vi "XImc Example One axis.vi"() -> ()   [LabVIEW 2017]
uses:
  subvi/XImc Example 1 CS.ctl
  libximc.lvlib
panel:
  in  "?":enum32{"Move settings"}(tab)
  in  "Speed":i32
  in  "GMOV":bool
  in  "SMOV":bool
  in  "Accel":i32
  in  "Decel":i32
  in  "Antiplay":i32
  out "Speed":dbl format="%#.2f"
  out "Accel":i16
  out "Decel":i16 format="%#.2f"
  out "Antiplay":i32
  out "Speed":dbl format="%#.2f steps/s"
  out "Temperature":dbl format="%#.2f C"
  out "USB current":dbl format="%#.2f mA"
  out "USB voltage":dbl format="%#.2f V"
  out "Power current":dbl format="%#.2f mA"
  out "Power voltage":dbl format="%#.2f V"
  in  "Stop motion":bool
  in  "ZEROCOMM":bool
  in  "HOME":bool
  in  "RIGHT":bool
  in  "LEFT":bool
  out "controller serial number":u32
  out "function return":i32
  out "Id":i32
  in  "SSTP":bool
  in  "Shift on":bool
  in  "?":i32
  in  "Move to":bool
  in  "?":i32
  out "?":dbl format="%#.2f"
  in  "Controller":u16(ring) items=["xi-com:\\\\.\\COM4"]
  in  "Find controllers":bool
  in  "Close application":bool
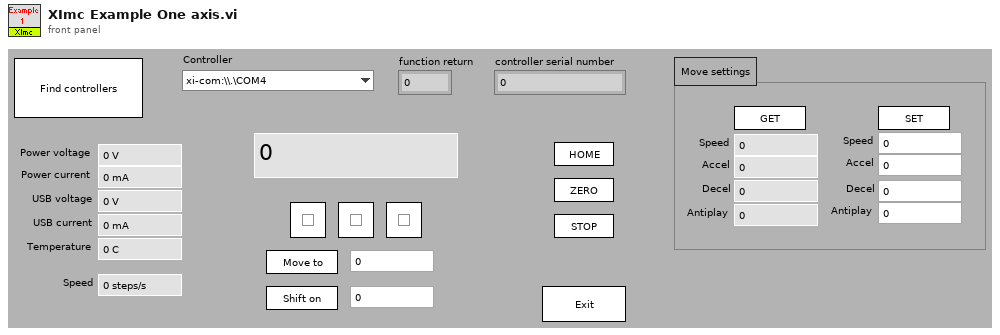
[diagram p1: front panel]
types:
  T1 = typedef "XImc Example 1 CS.ctl" = enum16{"Initialize_App", "Idle", "Find_Controllers", "Initialize_Controller", "Set_Parameters", "Get_Status", "Start_Motion", "Move_Relative", "Stop_Motion", "ZEROCOMM", "HOME", "LEFT", "RIGT", "SSTP", "Close_Controller", "Error_Handler", "Close_App", "Get_Move_Settings", "Set_Move_Settings"}
  T2 = cluster{"enumeration":i32, "Number of controllers":i32, "Controller name":string[], "variant":variant, "quit":bool, "Id":i32}
  T3 = cluster{"MoveSts":u32, "MvCmdSts":u32, "PWRSts":u32, "EncSts":u32, "WindSts":u32, "CurPosition":i32, "uCurPosition":i32, "@dummy control@":i8, "@dummy control@":i8, "@dummy control@":i8, "@dummy control@":i8, "EncPosition":i64, "CurSpeed":i32, "uCurSpeed":i32, "Ipwr":i32, "Upwr":i32, "Iusb":i32, "Uusb":i32, "CurT":i32, "Flags":u32, "GPIOFlags":u32, "CmdBufFreeSpace":u32}
  T4 = cluster{"Speed":u32, "uSpeed":u32, "Accel":u32, "Decel":u32, "AntiplaySpeed":u32, "uAntiplaySpeed":u32}
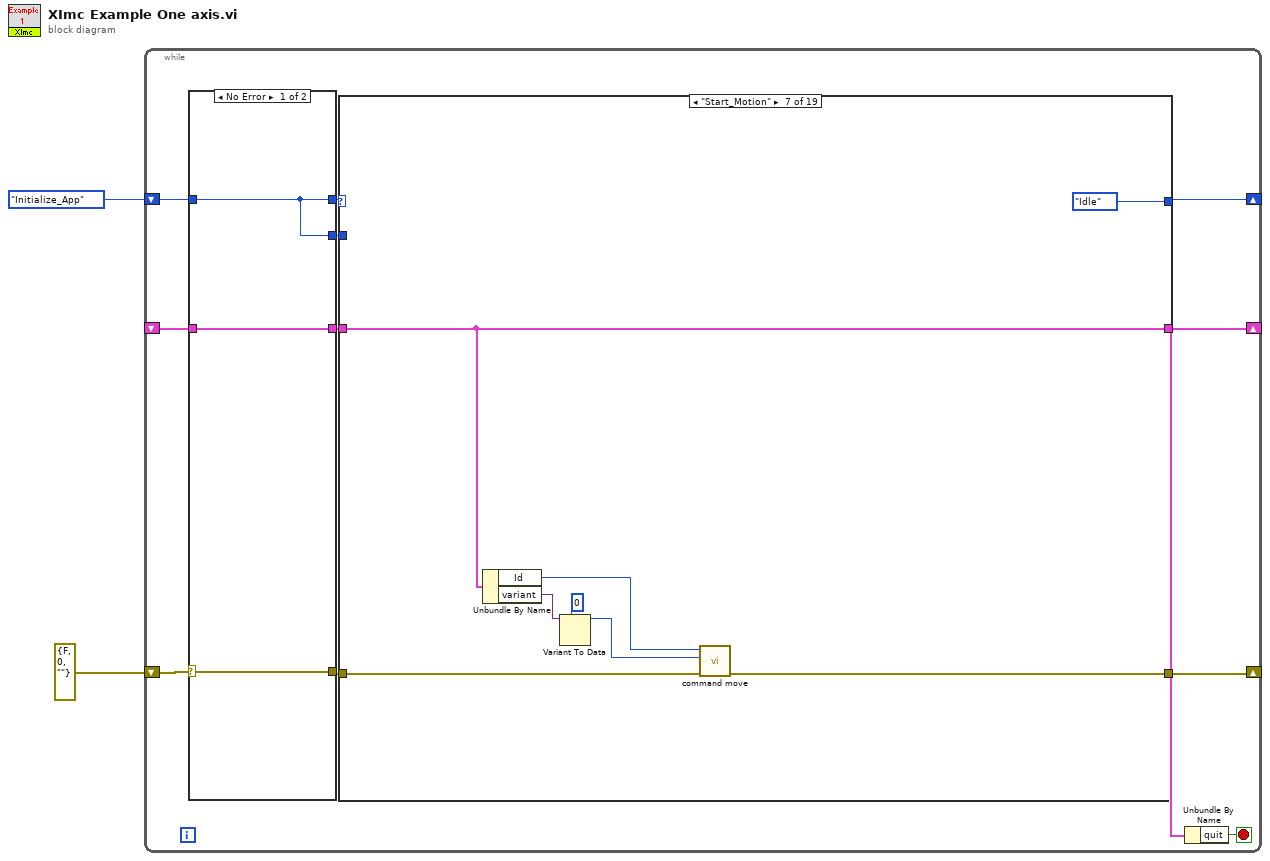
[diagram p0: block diagram]
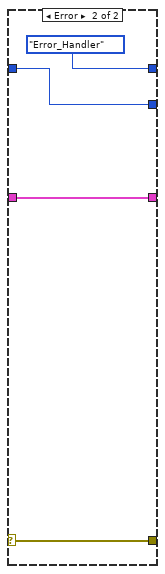
[diagram p2: hidden frame]
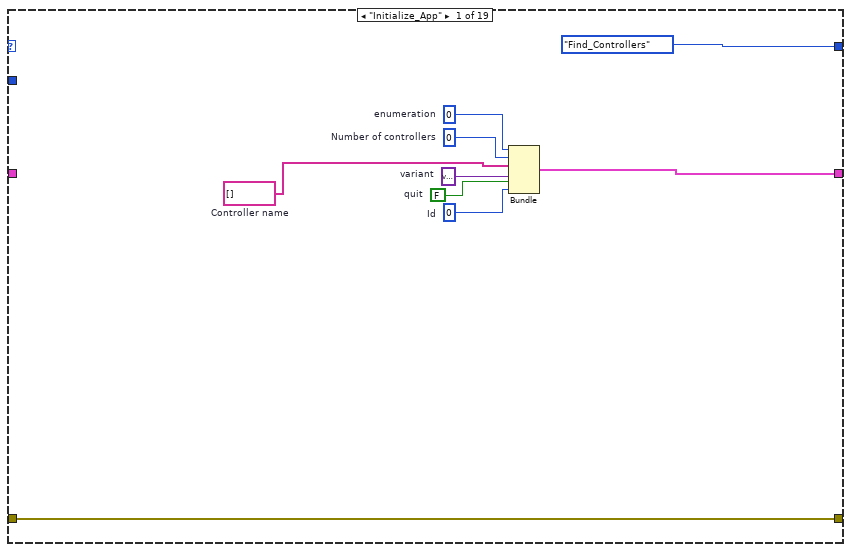
[diagram p3: hidden frame]
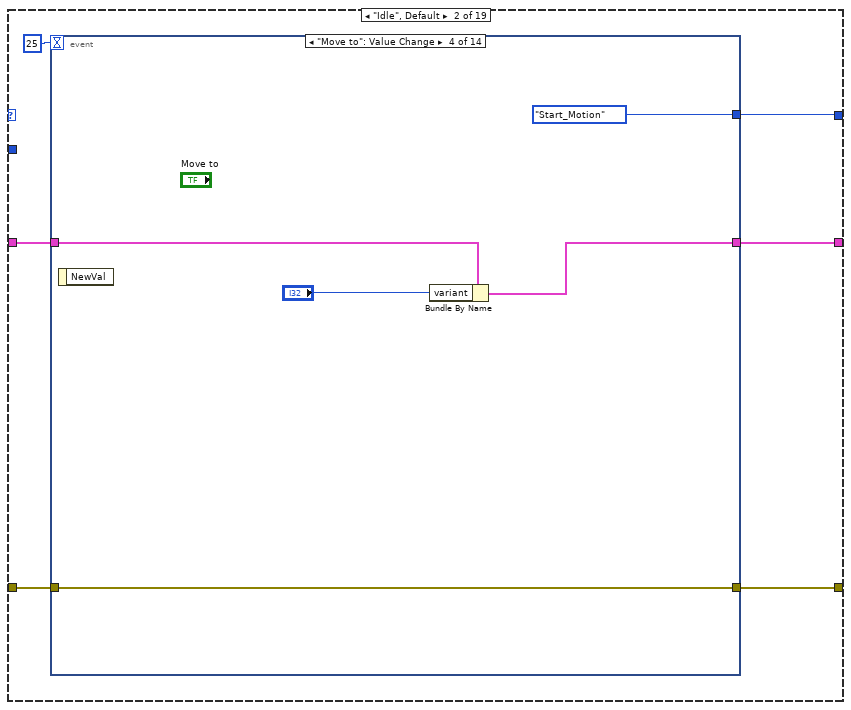
[diagram p4: hidden frame]
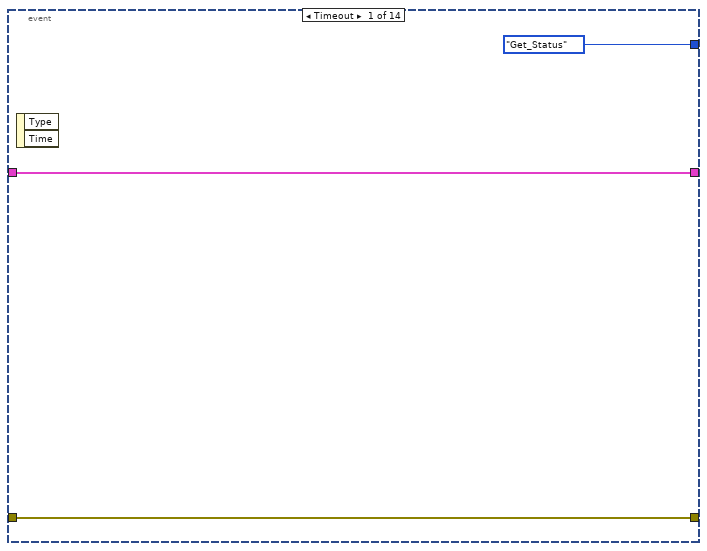
[diagram p5: hidden frame]
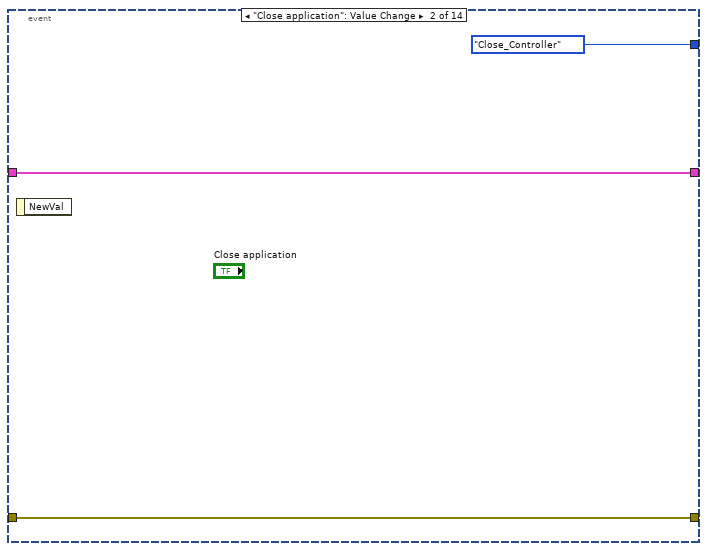
[diagram p6: hidden frame]
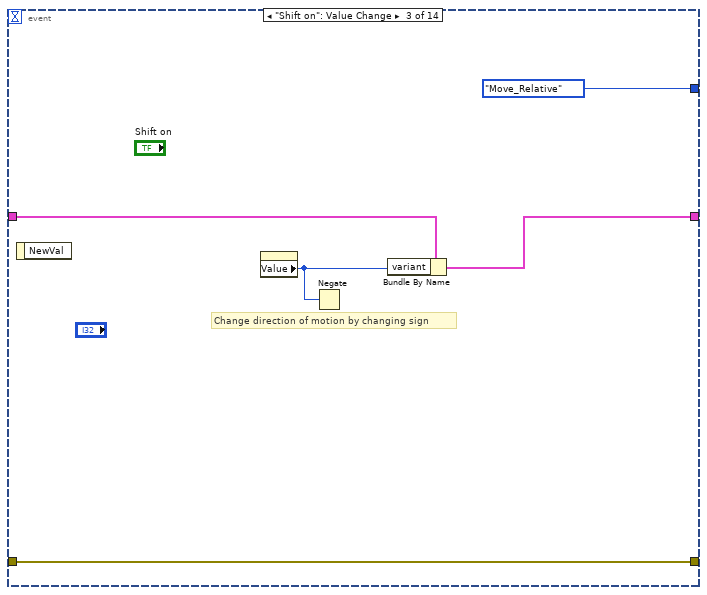
[diagram p7: hidden frame]
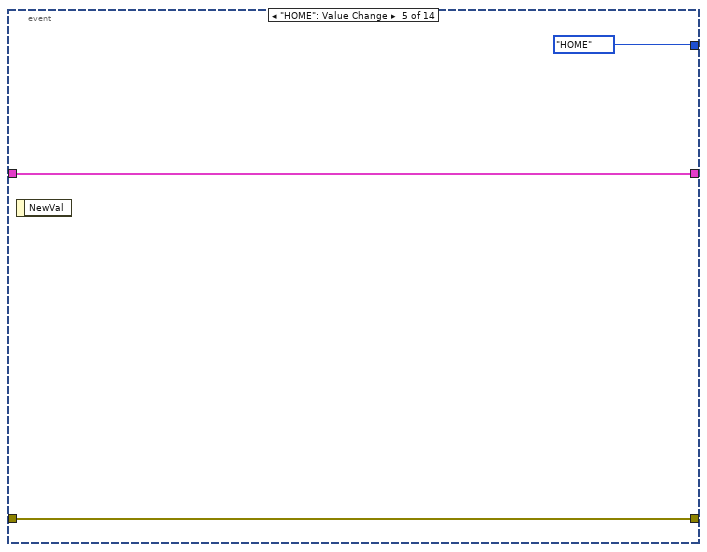
[diagram p8: hidden frame]
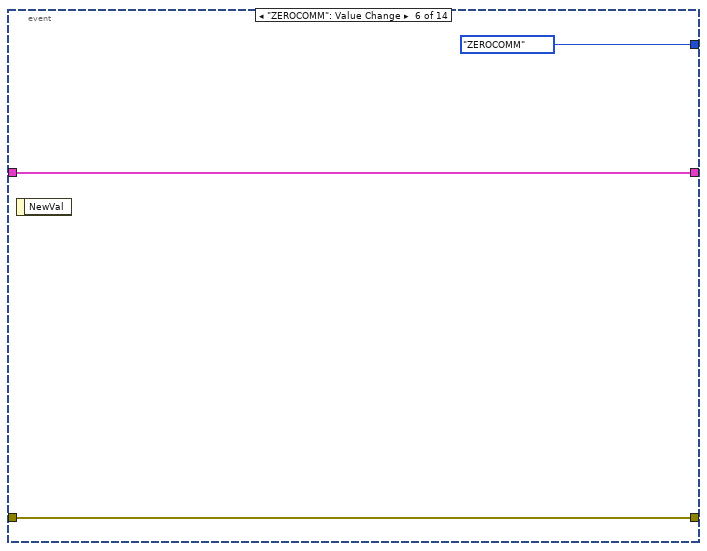
[diagram p9: hidden frame]
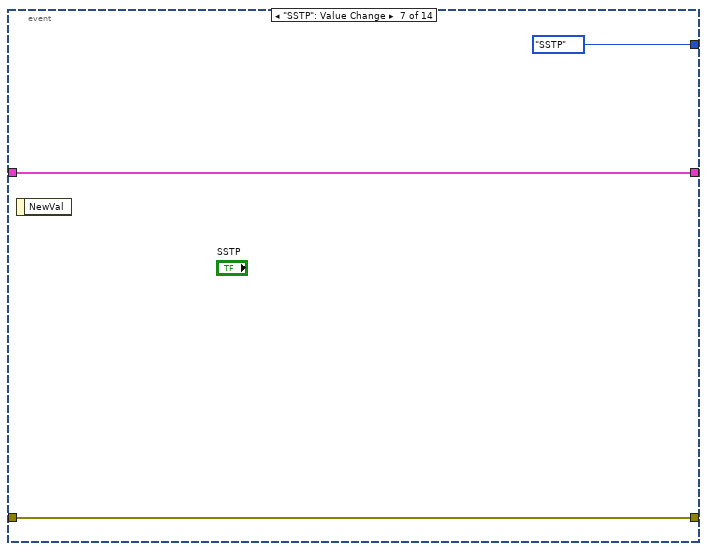
[diagram p10: hidden frame]
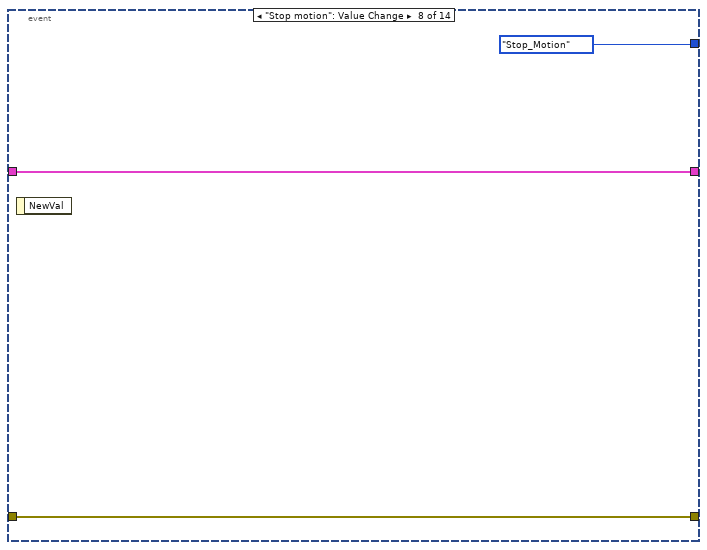
[diagram p11: hidden frame]
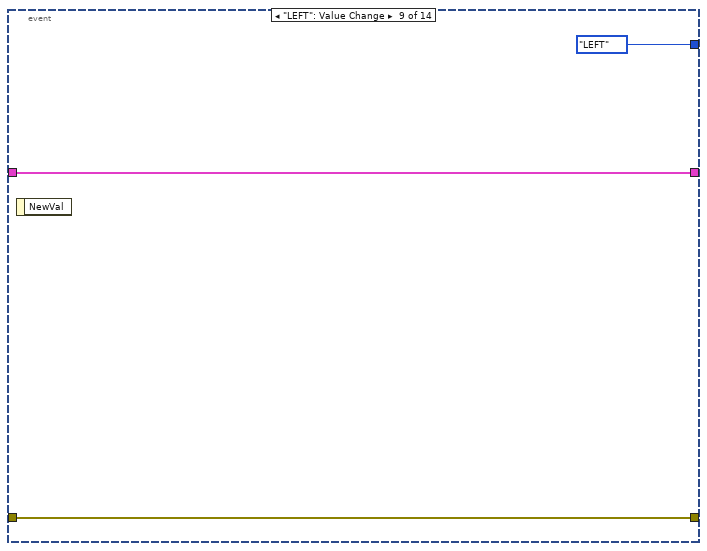
[diagram p12: hidden frame]
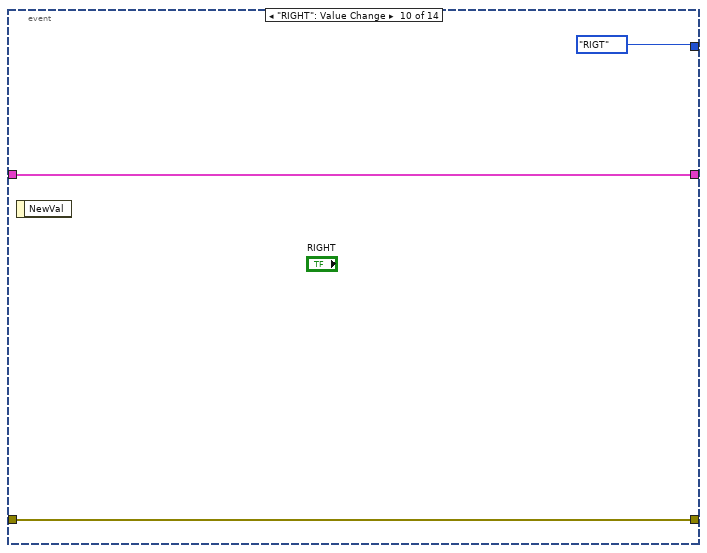
[diagram p13: hidden frame]
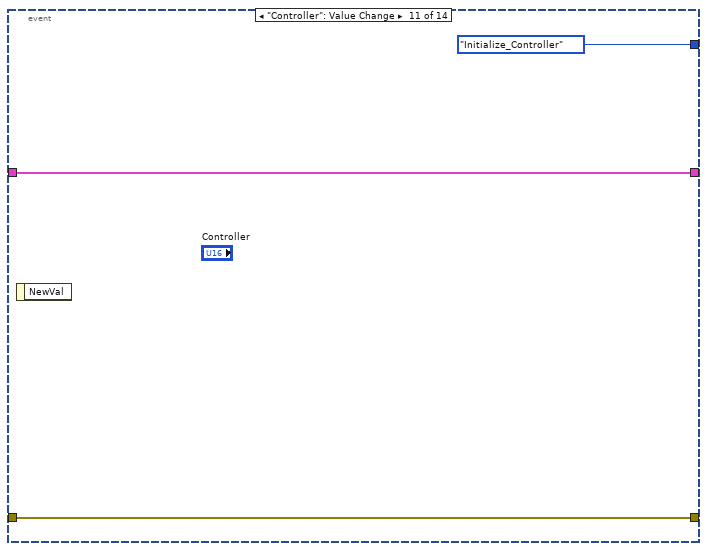
[diagram p14: hidden frame]
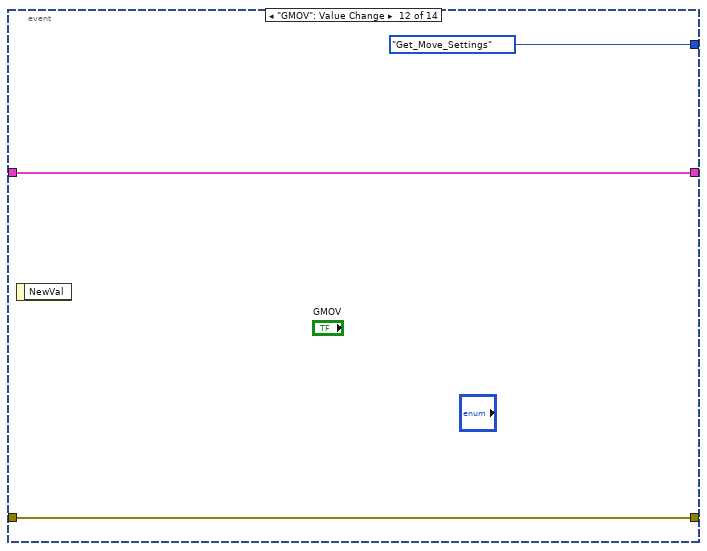
[diagram p15: hidden frame]
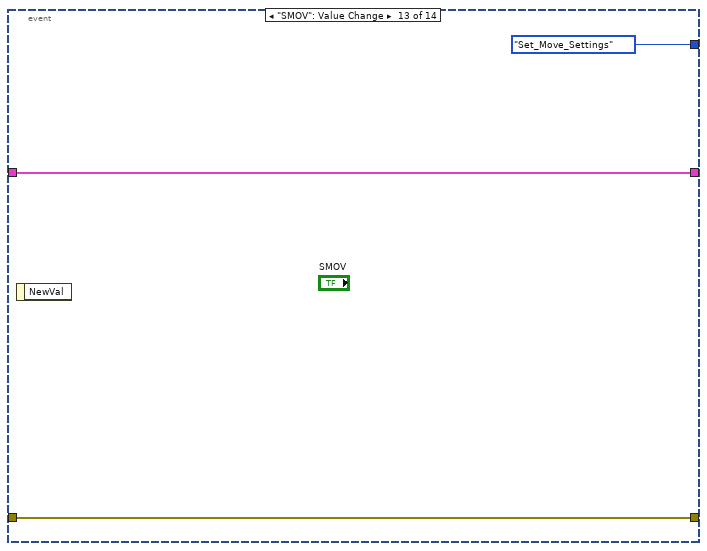
[diagram p16: hidden frame]
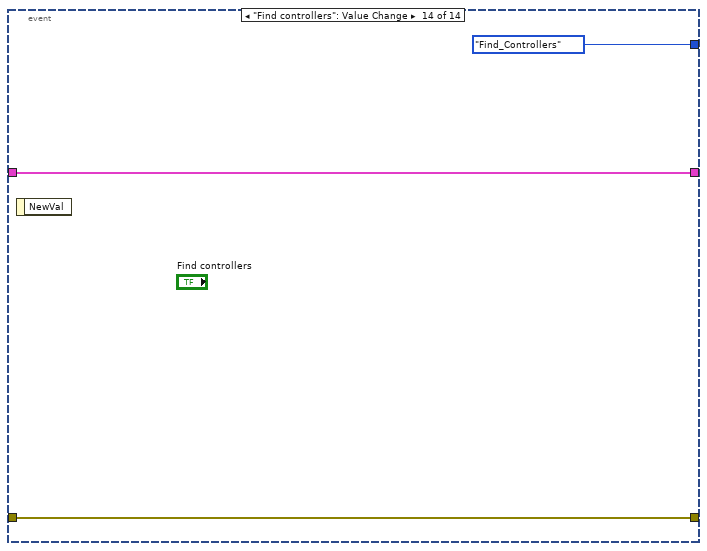
[diagram p17: hidden frame]
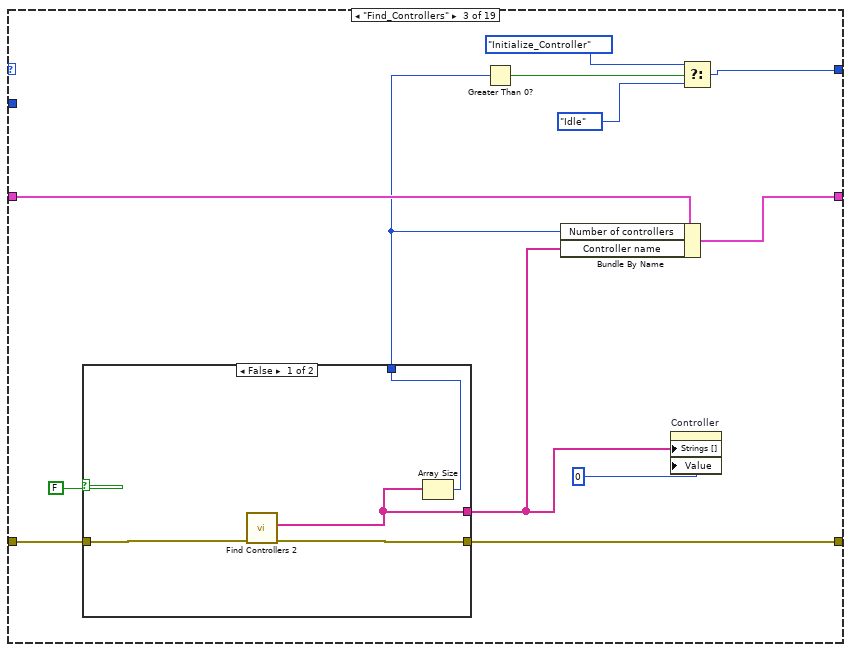
[diagram p18: hidden frame]
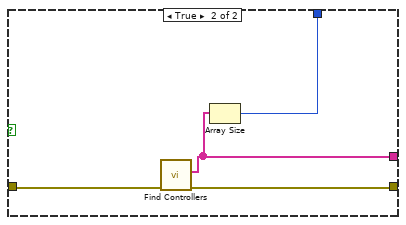
[diagram p19: hidden frame]
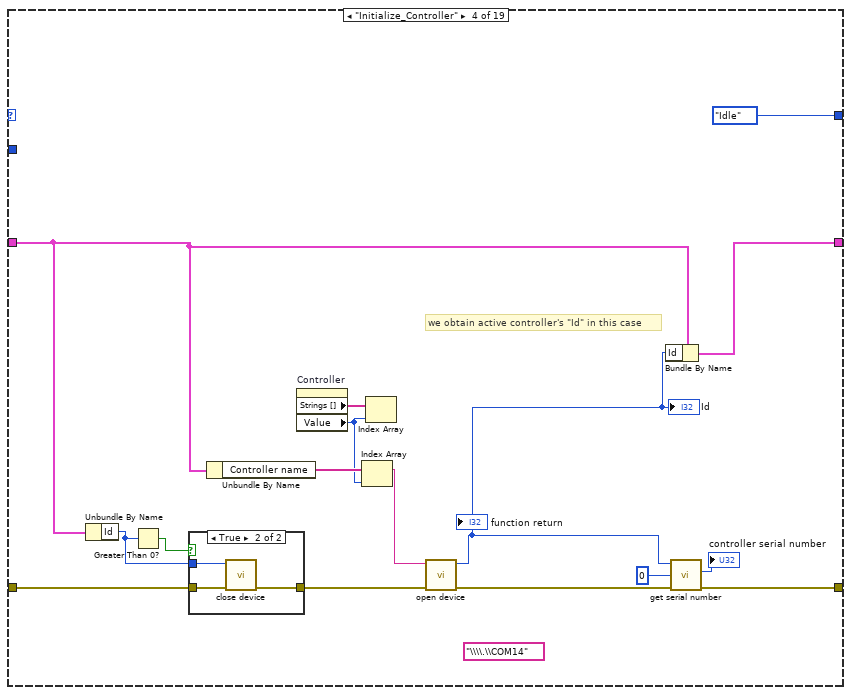
[diagram p20: hidden frame]
diagram:
  n1 = while {
    shift-right: [w13] -> _
    shift-left: XImc_Example_1_CS."Initialize_App" ("Case") -> [w6]
    shift-right: [w12] -> _
    shift-left: _ -> [w8]
    shift-right: [w3] -> _
    shift-left: errorcluster {"status"=FALSE, "code"=0, "source"=""} ("error in (no error)") -> [w10]
    stop <- w11 stop-if-true
    n2 = case shown="No Error" w10 {
      selector: w10 -> [w16 w19]
      tunnel: [w16 w19] -> w9
      tunnel: w8 -> [w15 w17]
      tunnel: [w15 w17] -> w7
      tunnel: w6 -> [w14 w18]
      tunnel: [w14 XImc_Example_1_CS."Error_Handler" ("Case")] -> w5
      tunnel: [w14 w18] -> w4
      frame No Error {
      }
      frame Error {
      }
    }
    n3 = case shown="\"Start_Motion\"" w5 {
      tunnel: [XImc_Example_1_CS."Find_Controllers" ("Case") w33 w91 XImc_Example_1_CS."Idle" ("Case") XImc_Example_1_CS."Idle" ("Case") XImc_Example_1_CS."Idle" ("Case") XImc_Example_1_CS."Idle" ("Case") XImc_Example_1_CS."Idle" ("Case") XImc_Example_1_CS."Idle" ("Case") XImc_Example_1_CS."Idle" ("Case") XImc_Example_1_CS."Idle" ("Case") XImc_Example_1_CS."Idle" ("Case") XImc_Example_1_CS."Idle" ("Case") XImc_Example_1_CS."Idle" ("Case") XImc_Example_1_CS."Idle" ("Case") XImc_Example_1_CS."Idle" ("Case") XImc_Example_1_CS."Close_App" ("Case") w224 XImc_Example_1_CS."Idle" ("Case")] -> w13
      tunnel: [w26 w32 w88 w115 w123 w141 w151 w159 w164 w166 w174 w179 w181 w189 w191 w211 w216 w223 w226] -> w12
      tunnel: w9 -> [w25 w35 w87 w108 w122 w143 w148 w156 w163 w169 w172 w177 w183 w187 w196 w209 w214 w222 w229]
      tunnel: w7 -> [_ w31 w89 w110 w123 w141 w151 w159 w164 w166 w174 w179 w181 w189 w191 w211 w216 w223 w227]
      tunnel: w4 -> [_ _ _ _ _ _ _ _ _ _ _ _ _ _ _ _ _ w224 _]
      tunnel: [w25 w30 w86 w111 w122 w142 w147 w155 w161 w168 w171 w176 w182 w186 w198 w207 w217 w221 w229] -> w3
      frame "Initialize_App" {
        w21 = string[] []  # Controller name
        w22 = 0  # enumeration
        w23 = 0  # Number of controllers
        w24 = 0  # Id
        w27 = FALSE  # quit
        w28 = variant  # variant
        n4 = Bundle("enumeration"=w22, "Number of controllers"=w23, "Controller name"=w21, "variant"=w28, "quit"=w27, "Id"=w24) -> (w26:T2)  [unwired: 1 in]
      }
      frame "Idle", Default {
        n5 = event shown="[3] \"Move to\": Value Change" {
          selector: _ -> [_ _ _ _ _ _ _ _ _ _ _ _ _ _]
          dyn-events: _ -> [_ _ _ _ _ _ _ _ _ _ _ _ _ _]
          timeout: 25 -> [_ _ _ _ _ _ _ _ _ _ _ _ _ _]
          tunnel: w35 -> [w36 w39 w45 w50 w53 w56 w59 w61 w65 w68 w71 w75 w76 w79]
          tunnel: [XImc_Example_1_CS."Get_Status" ("Case") XImc_Example_1_CS."Close_Controller" ("Case") XImc_Example_1_CS."Move_Relative" ("Case") XImc_Example_1_CS."Start_Motion" ("Case") XImc_Example_1_CS."HOME" ("Case") XImc_Example_1_CS."ZEROCOMM" ("Case") XImc_Example_1_CS."SSTP" ("Case") XImc_Example_1_CS."Stop_Motion" ("Case") XImc_Example_1_CS."LEFT" ("Case") XImc_Example_1_CS."RIGT" ("Case") XImc_Example_1_CS."Initialize_Controller" ("Case") XImc_Example_1_CS."Get_Move_Settings" ("Case") XImc_Example_1_CS."Set_Move_Settings" ("Case") XImc_Example_1_CS."Find_Controllers" ("Case")] -> w33
          tunnel: [w37 w40 w43 w48 w54 w57 w58 w62 w66 w69 w70 w73 w77 w80] -> w32
          tunnel: w31 -> [w37 w40 w44 w49 w54 w57 w58 w62 w66 w69 w70 w73 w77 w80]
          tunnel: [w36 w39 w45 w50 w53 w56 w59 w61 w65 w68 w71 w75 w76 w79] -> w30
          event Timeout {
            n6 = event-data() -> ()  [unwired: 1 in, 2 out]
          }
          event "Close application": Value Change {
            n7 = event-data() -> ()  [unwired: 1 in, 1 out]
          }
          event "Shift on": Value Change {
            # "Change direction of motion by changing sign"
            n8 = event-data() -> ()  [unwired: 1 in, 1 out]
            n9 = property class="DigNum (strict)"() -> ("Value"=w42:i32)  [unwired: 2 in, 2 out]
            n10 = Negate(x=w42) -> ()  [unwired: 1 out]
            n11 = Bundle By Name(cluster=w44, "variant"=w42) -> (w43:T2)
          }
          event "Move to": Value Change {
            n12 = event-data() -> ()  [unwired: 1 in, 1 out]
            n13 = Bundle By Name(cluster=w49, "variant"="?") -> (w48:T2)
          }
          event "HOME": Value Change {
            n14 = event-data() -> ()  [unwired: 1 in, 1 out]
          }
          event "ZEROCOMM": Value Change {
            n15 = event-data() -> ()  [unwired: 1 in, 1 out]
          }
          event "SSTP": Value Change {
            n16 = event-data() -> ()  [unwired: 1 in, 1 out]
          }
          event "Stop motion": Value Change {
            n17 = event-data() -> ()  [unwired: 1 in, 1 out]
          }
          event "LEFT": Value Change {
            n18 = event-data() -> ()  [unwired: 1 in, 1 out]
          }
          event "RIGHT": Value Change {
            n19 = event-data() -> ()  [unwired: 1 in, 1 out]
          }
          event "Controller": Value Change {
            n20 = event-data() -> ()  [unwired: 1 in, 1 out]
          }
          event "GMOV": Value Change {
            n21 = event-data() -> ()  [unwired: 1 in, 1 out]
          }
          event "SMOV": Value Change {
            n22 = event-data() -> ()  [unwired: 1 in, 1 out]
          }
          event "Find controllers": Value Change {
            n23 = event-data() -> ()  [unwired: 1 in, 1 out]
          }
        }
      }
      frame "Find_Controllers" {
        n24 = case shown="False" FALSE {
          tunnel: w87 -> [w96 w101]
          tunnel: [w97 w100] -> w86
          tunnel: [w94 w98] -> w85
          tunnel: [w95 w99] -> w82
          frame False {
            n25 = call "Find Controllers 2.vi"("error in (no error)"=w96) -> ("error out"=w97:errorcluster, "Names"=w95:string[])  [unwired: 9 in]
            n26 = Array Size(array=w95) -> (size(s)=w94:i32)
          }
          frame True {
            n27 = call "Find Controllers.vi"("error in (no error)"=w101) -> ("error out"=w100:errorcluster, "Controllers"=w99:string[])  [unwired: 8 in, 1 out]
            n28 = Array Size(array=w99) -> (size(s)=w98:i32)
          }
        }
        n29 = Greater Than 0?(x=w85) -> (x > 0?=w93:bool)
        n30 = Bundle By Name(cluster=w89, "Number of controllers"=w85, "Controller name"=w82) -> (w88:T2)
        n31 = property on="Controller" class="Ring (strict)"("Strings []"=w82, "Value"=0) -> ()  [unwired: 2 in, 2 out]
        n32 = Select(t=XImc_Example_1_CS."Initialize_Controller", s=w93, f=XImc_Example_1_CS."Idle" ("Case")) -> (s? t:f=w91:T1)
      }
      frame "Initialize_Controller" {
        (unwired) "\\\\.\\COM14" ("name")
        # "we obtain active controller's \"Id\" in this case"
        n33 = Unbundle By Name(w110) -> ("Id"=w109:i32)
        n34 = Greater Than 0?(x=w109) -> (x > 0?=w106:bool)
        n35 = case shown="True" w106 {
          tunnel: w109 -> [_ w121]
          tunnel: w108 -> [w118 w120]
          tunnel: [w118 w119] -> w107
          frame False {
          }
          frame True {
            n36 = call "close device.vi"("error in (no error)"=w120, "id"=w121) -> ("error out"=w119:errorcluster)  [unwired: 7 in, 2 out]
          }
        }
        n37 = Unbundle By Name(w110) -> ("Controller name"=w112:string[])
        n38 = property on="Controller" class="Ring (strict)"() -> ("Strings []"=w116:string[], "Value"=w104:u16)  [unwired: 2 in, 2 out]
        n39 = Index Array(array=w112, index=w104) -> (element=w105:string)
        n40 = Index Array(array=w116, index=w104) -> ()  [unwired: 1 out]
        n41 = call "open device.vi"("error in (no error)"=w107, "name"=w105) -> ("error out"=w103:errorcluster, "function return"=w102:i32)  [unwired: 8 in]
        "Id" <- w102
        "function return" <- w102
        n42 = Bundle By Name(cluster=w110, "Id"=w102) -> (w115:T2)
        n43 = call "get serial number.vi"("error in (no error)"=w103, "SerialNumber"=u32 0 ("serial"), "id"=w102) -> ("error out"=w111:errorcluster, "SerialNumber out"=→"controller serial number":u32)  [unwired: 6 in, 1 out]
      }
      frame "Set_Parameters" {
      }
      frame "Get_Status" {
        n44 = Unbundle By Name(w141) -> ("Id"=w140:i32)
        n45 = call "get status.vi"("error in (no error)"=w143, "id"=w140) -> ("error out"=w142:errorcluster, "status out"=w138:T3, "function return"=w139:i32)  [unwired: 7 in]
        n46 = Greater Or Equal To 0?(x=w139) -> ()  [unwired: 1 out]
        n47 = Unbundle By Name(w138) -> ("Upwr"=w133:i32, "Ipwr"=→"Power current":i32, "Uusb"=w131:i32, "Iusb"=→"USB current":i32, "CurT"=w127:i32, "CurSpeed"=→"Speed":i32, "CurPosition"=→"?":i32)  [unwired: 3 out]
        n48 = Multiply(x=0.01, y=w133) -> (x*y=→"Power voltage":dbl)
        n49 = Multiply(x=0.1, y=w127) -> (x*y=→"Temperature":dbl)
        n50 = Multiply(x=w131, y=0.01) -> (x*y=→"USB voltage":dbl)
      }
      frame "Start_Motion" {
        n51 = Unbundle By Name(w151) -> ("Id"=w145:i32, "variant"=w150:variant)
        n52 = Variant To Data(type=u32 0, Variant=w150) -> (data=w146:u32)  [unwired: 1 in, 1 out]
        n53 = call "command move.vi"("error in (no error)"=w148, "Position"=w146, "id"=w145) -> ("error out"=w147:errorcluster)  [unwired: 7 in, 1 out]
      }
      frame "Move_Relative" {
        n54 = Unbundle By Name(w159) -> ("Id"=w153:i32, "variant"=w158:variant)
        n55 = Variant To Data(type=0, Variant=w158) -> (data=w154:i32)  [unwired: 1 in, 1 out]
        n56 = call "command movr.vi"("error in (no error)"=w156, "DeltaPosition"=w154, "id"=w153) -> ("error out"=w155:errorcluster)  [unwired: 7 in, 1 out]
      }
      frame "Stop_Motion" {
        n57 = Unbundle By Name(w164) -> ("Id"=w162:i32)
        n58 = call "command stop.vi"("error in (no error)"=w163, "id"=w162) -> ("error out"=w161:errorcluster)  [unwired: 8 in, 1 out]
      }
      frame "SSTP" {
        n59 = Unbundle By Name(w166) -> ("Id"=w167:i32)
        n60 = call "command sstp.vi"("error in (no error)"=w169, "id"=w167) -> ("error out"=w168:errorcluster)  [unwired: 8 in, 1 out]
      }
      frame "LEFT" {
        n61 = Unbundle By Name(w174) -> ("Id"=w173:i32)
        n62 = call "command left.vi"("error in (no error)"=w172, "id"=w173) -> ("error out"=w171:errorcluster)  [unwired: 8 in, 1 out]
      }
      frame "RIGT" {
        n63 = Unbundle By Name(w179) -> ("Id"=w178:i32)
        n64 = call "command right.vi"("error in (no error)"=w177, "id"=w178) -> ("error out"=w176:errorcluster)  [unwired: 8 in, 1 out]
      }
      frame "HOME" {
        n65 = Unbundle By Name(w181) -> ("Id"=w184:i32)
        n66 = call "command home.vi"("error in (no error)"=w183, "id"=w184) -> ("error out"=w182:errorcluster)  [unwired: 8 in, 1 out]
      }
      frame "ZEROCOMM" {
        n67 = Unbundle By Name(w189) -> ("Id"=w188:i32)
        n68 = call "command zero.vi"("error in (no error)"=w187, "id"=w188) -> ("error out"=w186:errorcluster)  [unwired: 8 in, 1 out]
      }
      frame "Get_Move_Settings" {
        n69 = Unbundle By Name(w191) -> ("Id"=w199:i32)
        n70 = call "get move settings.vi"("error in (no error)"=w196, "id"=w199) -> ("error out"=w198:errorcluster, "move_settings out"=w197:T4)  [unwired: 7 in, 1 out]
        n71 = Unbundle By Name(w197) -> ("Speed"=→"Speed":u32, "Accel"=→"Accel":u32, "Decel"=→"Decel":u32, "AntiplaySpeed"=→"Antiplay":u32)  [unwired: 2 out]
      }
      frame "Set_Move_Settings" {
        n72 = call "get move settings.vi"() -> ("move_settings out"=w205:T4)  [unwired: 9 in, 2 out]
        n73 = Bundle(cluster=w205, "Speed"="Speed", "Accel"="Accel", "Decel"="Decel", "AntiplaySpeed"="Antiplay") -> (w206:T4)  [unwired: 2 in]
        n74 = Variant To Data(error in=w209, type=w205, Variant=w206) -> (data=w210:T4, error out=w208:errorcluster)
        n75 = Unbundle By Name(w211) -> ("Id"=w212:i32)
        n76 = call "set move settings.vi"("error in (no error)"=w208, "move_settings"=w210, "id"=w212) -> ("error out"=w207:errorcluster)  [unwired: 7 in, 1 out]
      }
      frame "Close_Controller" {
        n77 = Unbundle By Name(w216) -> ("Id"=w219:i32)
        n78 = call "close device.vi"("error in (no error)"=w214, "id"=w219) -> ("error out"=w218:errorcluster)  [unwired: 7 in, 2 out]
        n79 = Unbundle By Name(w216) -> ("enumeration"=w215:i32)  [unwired: 1 out]
        n80 = call "free enumerate devices.vi"("error in (no error)"=w218, "device_enumeration"=w215) -> ("error out"=w217:errorcluster)  [unwired: 8 in, 1 out]
      }
      frame "Error_Handler" {
        # "here we return to the last case before error occured"
        n81 = call <vilib>:"Clear Errors.vi"("error in (no error)"=w222) -> ("error out"=w221:errorcluster)  [unwired: 5 in, 1 out]
      }
      frame "Close_App" {
        n82 = Bundle By Name(cluster=w227, "quit"=TRUE) -> (w226:T2)
      }
    }
    n83 = Unbundle By Name(w12) -> ("quit"=w11:bool)
  }
